vi "Test_2.vi"() -> ()   [LabVIEW 2018]
panel:
  in  "Log File Input":T1={"Log File Input"="TECH", "Log Entry Type"=enum."WARNING"}
  in  "milliseconds to wait":u32=100
  in  "stop":bool
  out "error out":errorcluster
  in  "error in (no error)":errorcluster
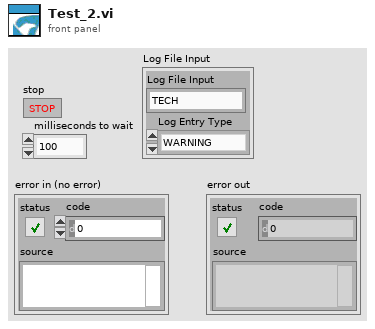
[diagram p1: front panel]
types:
  T1 = cluster{"Log File Input":string, "Log Entry Type":enum16{"STANDARD", "WARNING", "CRITICAL"}}
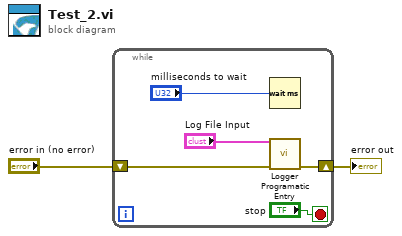
[diagram p0: block diagram]
diagram:
  n1 = while {
    shift-right: [w7] -> w2
    shift-left: "error in (no error)" -> [w5]
    stop <- "stop" stop-if-true
    n2 = Wait (ms)(milliseconds to wait="milliseconds to wait") -> ()  [unwired: 1 out]
    n3 = call "Logger Programatic Entry.vi"("Log File Input"="Log File Input", "error in (no error)"=w5) -> ("error out"=w7:errorcluster)  [unwired: 13 in]
  }
  "error out" <- w2
